vi "All Created Queues.vi"(9 "Priority?":bool, 10 "Msg Strategy":refnum<class "Msg Strategy.lvclass">, 11 "Template Queue in":refnum<class "Template Queue.lvclass">) -> (3 "Template Queue out":refnum<class "Template Queue.lvclass">)   [LabVIEW 2021, in "_Template.lvlib" / "Templates.lvlib" / "Template Queue.lvlib" / "Template Queue.lvclass"]
uses:
  Template Queue.lvclass
  <vilib>/jettl/jettl/jettl/Msg Strategy/Msg Strategy.lvclass
  Template Queue.lvclass/Template Queue.ctl
  <vilib>/jettl/jettl/jettl/Queue/Queue.lvclass
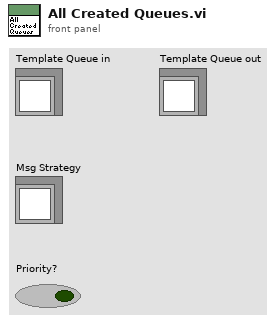
[diagram p1: front panel]
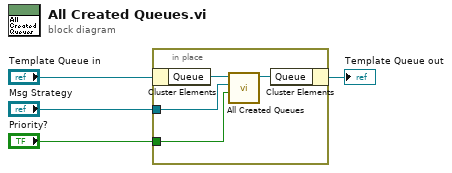
[diagram p0: block diagram]
diagram:
  n1 = in-place {
    in-place-border: "Msg Strategy" -> [w6]
    in-place-border: "Priority?" -> [w5]
    n2 = in-place-cluster #1("Template Queue in") -> ("Queue"=w8:refnum<class "Queue.lvclass">)
    n3 = call-dynamic "All Created Queues.vi"("Priority?"=w5, "Msg Strategy"=w6, "Queue in"=w8) -> ("Queue out"=w7:refnum<class "Queue.lvclass">)  [unwired: 8 in]
    n4 = in-place-cluster #1("Queue"=w7) -> (→"Template Queue out":refnum<class "Template Queue.lvclass">)
  }
